vi "Log Data.vi"(8 "error in (no error)":T1 caption="entrée d'erreur (pas d'erreur)", 10 "File d'attente de données":refnum<queue>, 11 "Configuration de l'enregistrement":T2) -> (0 "error out":T1 caption="sortie d'erreur")   [LabVIEW 2018, in "Logging.lvlib"]
doc: "Ce VI utilise la fonction TDMS - Écrire pour écrire des données dans un fichier TDMS."
uses:
  Logging.lvlib
  Logging Configuration.ctl
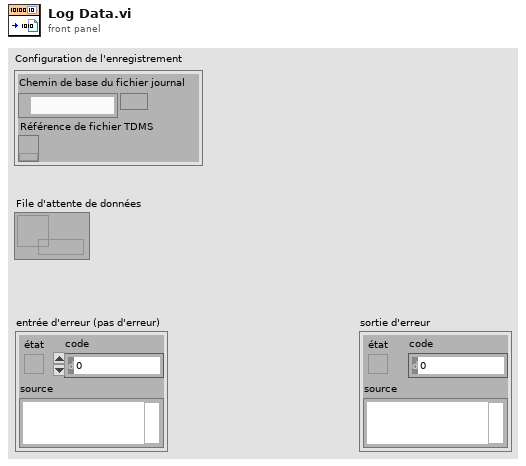
[diagram p1: front panel]
types:
  T1 = cluster{"état":bool, "code":i32, "source":string}
  T2 = typedef "Logging.lvlib/Logging Configuration.ctl" = cluster{"Chemin de base du fichier journal":path, "Référence de fichier TDMS":refnum<k34>}
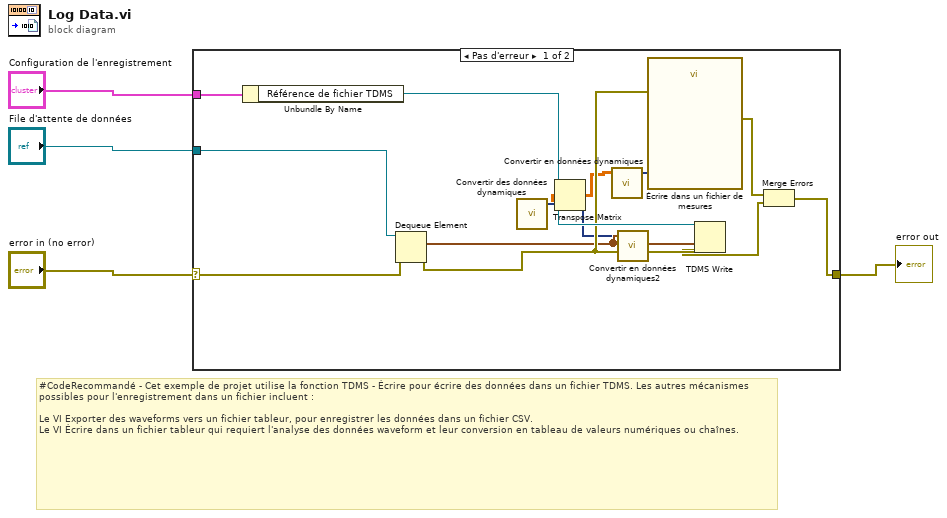
[diagram p0: block diagram]
diagram:
  # "#CodeRecommandé - Cet exemple de projet utilise la fonction TDMS - Écrire pour écrire des données dans un fichier TDMS. Les autres mécanismes possibles pour l'enregistrement dans un fichier incluent :\n\nLe VI Exporter des waveforms vers un fichier tableur, pour enregistrer les données dans un fichier CSV.\nLe VI Écrire dans un fichier tableur qui requiert l'analyse des données waveform et leur conversion en tableau de valeurs numériques ou chaînes."
  n1 = case shown="Pas d'erreur" "error in (no error)" {
    selector: "error in (no error)" -> [w16 w18]
    tunnel: "Configuration de l'enregistrement" -> [w17 _]
    tunnel: "File d'attente de données" -> [w15 _]
    tunnel: [w10 w18] -> w2
    frame No Error {
      n2 = Unbundle By Name(w17) -> ("Référence de fichier TDMS"=w14:refnum<k34>)
      n3 = Dequeue Element(queue=w15, error in (no error)=w16) -> (element=w7:waveform(dbl)[], error out=w13:errorcluster)  [unwired: 1 in, 2 out]
      n4 = call "Convertir en données dynamiques2"("Array of Waveforms"=w7) -> ("Dynamic Data Type"=w6:dynamicdata)  [unwired: 3 in]
      n5 = call "Convertir des données dynamiques"("Dynamic Data Type"=w6) -> ("Array"=w5:dbl[][])  [unwired: 3 in]
      n6 = Transpose Matrix(1:w5) -> (0:w9:dbl[][])
      n7 = call "Convertir en données dynamiques"("2D Array"=w9) -> ("Dynamic Data Type"=w8:dynamicdata)  [unwired: 3 in]
      n8 = call "Écrire dans un fichier de mesures"("Signals"=w8, "error in (no error)"=w13) -> ("error out"=w12:errorcluster)  [unwired: 15 in, 2 out]
      n9 = TDMS Write(0:w14, 9:w7, 11:w13) -> (15:w11:errorcluster)  [unwired: 3 in, 3 out]
      n10 = Merge Errors(w12, w11) -> (w10:errorcluster)
    }
    frame Error {
    }
  }
  "error out" <- w2
